vi "Initialize AI Task.vi"(8 "error in (no error)":errorcluster, 11 "BNT_DMQmx-MCSV-TC in":refnum<class "BNT_DAQmx-MCSV-RTD.lvclass">) -> (0 "error out":errorcluster, 3 "AI DAQmx Task":refnum<k21>)   [LabVIEW 2017, in "BNT_DAQmx.lvlib" / "BNT_DAQmx-MCSV-RTD.lvclass"]
doc: "Initialize DAQmx Analog Input task.\n\n<b>Default Implementation:</b> Analog Input Voltage\n\nThis dynamic dispatch VI can be overritten by derived classes to implement other analog input tasks."
uses:
  BNT_DAQmx-MCSV-RTD.lvclass
  C:/User/Brand/LVP/TASCA/UTCS/Packages/BNT_DAQmx/BNT_DAQmx-MCSV/BNT_DAQmx-MCSV.lvclass
  BNT_DAQmx-MCSV-RTD.lvclass/BNT_DAQmx-MCSV-RTD.ctl
  BNT_DAQmx-MCSV/BNT_DAQmx-MCSV.lvclass/BNT_DAQmx-MCSV.ctl
  Read Current Excitation Value.vi
  Read R0.vi
  Read Resistance Configuration.vi
  BNT_DAQmx-MCSV/Read AI Min.vi
  BNT_DAQmx-MCSV/Read AI Max.vi
  BNT_DAQmx-MCSV/Read AI DAQmx Physical Channels.vi
  Read Current Excitation Source.vi
  <vilib>/DAQmx/create/channels.llb/DAQmx Create Channel (AI-Temperature-RTD).vi
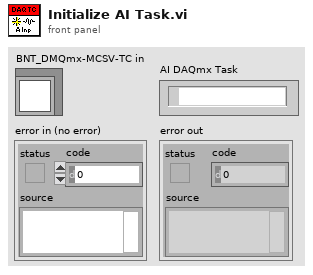
[diagram p1: front panel]
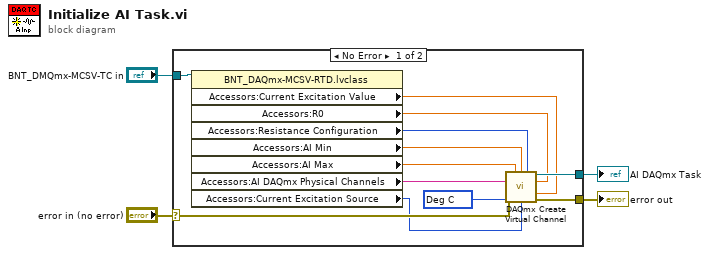
[diagram p0: block diagram]
diagram:
  n1 = case shown="No Error" "error in (no error)" {
    selector: "error in (no error)" -> [w16 w17]
    tunnel: [w15 w17] -> w3
    tunnel: "BNT_DMQmx-MCSV-TC in" -> [w13 _]
    tunnel: [w14 _] -> w1
    frame No Error {
      w9 = 10143 items=["Deg C"=10143, "Deg F"=10144, "Kelvins"=10325, "Deg R"=10145, "From Custom Scale"=10065] ("units")
      n2 = property class="BNT_DAQmx-MCSV-RTD.lvclass"(reference=w13) -> ("Accessors:Current Excitation Value"=w7:dbl, "Accessors:R0"=w8:dbl, "Accessors:Resistance Configuration"=w5:i32, "Accessors:AI Min"=w10:dbl, "Accessors:AI Max"=w11:dbl, "Accessors:AI DAQmx Physical Channels"=w12:tag, "Accessors:Current Excitation Source"=w6:i32)  [unwired: 1 in, 2 out]
      n3 = call-poly <vilib>:"DAQmx Create Virtual Channel.vi"("maximum value"=w11, "minimum value"=w10, "resistance configuration"=w5, "physical channels"=w12, "r0"=w8, "units"=w9, "current excitation value"=w7, "error in"=w16, "current excitation source"=w6) -> ("task out"=w14:refnum<k21>, "error out"=w15:errorcluster)  [unwired: 5 in]
    }
    frame Error {
    }
  }
  "error out" <- w3
  "AI DAQmx Task" <- w1
